vi "Commands.vi"(8 "error in (no error)":errorcluster, 11 "Node Ptr":T1 format="%.0x") -> (0 "error out":errorcluster)   [LabVIEW 2019, in "Diagnostics Addon System Explorer.lvlib"]
uses:
  Diagnostics Addon System Explorer.lvlib
  <vilib>/NI VeriStand/Custom Device API/Custom Device Item Ref.ctl
  Types/FG.Action.ctl
  Addon Shared/SubVIs/Constants.vi
  <vilib>/NI VeriStand/Custom Device API/NI VeriStand - Get Item Property.vi
  <vilib>/NI VeriStand/Custom Device API/Get Item Property (String).vi
  <vilib>/NI VeriStand/Custom Device API/Get Item Property (Variant).vi
  <vilib>/NI VeriStand/Custom Device API/Get Item Property (U32).vi
  <vilib>/NI VeriStand/Custom Device API/Get Item Property (Boolean).vi
  <vilib>/NI/NI VeriStand Advanced SysDef API/SysDef API/SysDef.Property.Set.vi
  <vilib>/NI/NI VeriStand Advanced SysDef API/_SubVIs/SysDef.Property.Set.String.vi
  <vilib>/NI/NI VeriStand Advanced SysDef API/_SubVIs/SysDef.Property.Set.Variant.vi
  <vilib>/NI/NI VeriStand Advanced SysDef API/_SubVIs/SysDef.Property.Set.U32.vi
  <vilib>/NI/NI VeriStand Advanced SysDef API/_SubVIs/SysDef.Property.Set.Boolean.vi
  <vilib>/NI VeriStand/Custom Device API/Custom Device API.lvlib
panel:
  in  "SHDocVw.IWebBrowser":refnum<k7>(container)
  in  "Header":cluster{"Section Name":string}={"Section Name"="Custom Device Item Settings"}
  in  "Description":string
  in  "Name":string
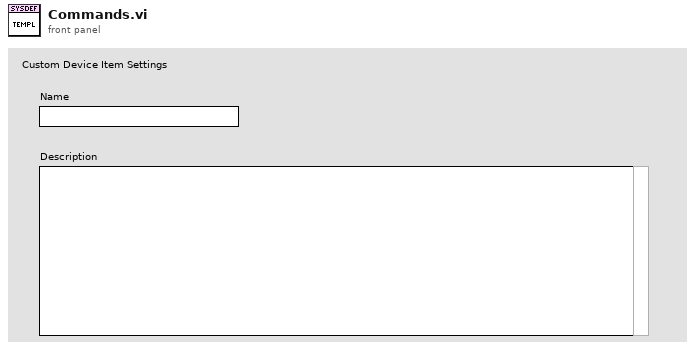
[diagram p1: front panel]
types:
  T1 = typedef "Custom Device API.lvlib/Custom Device Item Ref.ctl" = u64
  T2 = typedef "Diagnostics Addon System Explorer.lvlib/FG.Action.ctl" = enum16{"Get", "Set"}
  T3 = typedef "Diagnostics Addon Shared.lvlib/CAN.ctl" = cluster{"Interface":T4, "Baud Rate":u64, "Diagnostic Protocol":T5, "Transport Protocol":T6, "Transmit ID":u32, "Receive ID":u32, "Transmit Extension":u8, "Receive Extension":u8, "Receive UUDT ID":u32, "Enable Stream":bool, "VW TP Channel ID":u32, "Fill Frame":bool, "Fill Byte":u8, "Termination":bool, "LIN Cluster":refnum<k21>, "NAD":u8, "IO Mode":u32, "Max DLC":u16, "FD Baud Rate":u64, "Timeout":u32}
  T4 = typedef "Diagnostics Addon Shared.lvlib/CAN.Interface.ctl" = string
  T5 = typedef "Diagnostics Addon Shared.lvlib/Protocol.ctl" = enum16{"GMLAN", "KWP-2000", "UDS", "User-Defined"}
  T6 = typedef "Diagnostics Addon Shared.lvlib/Transport.ctl" = enum16{"ISO TP - Normal Mode", "ISO TP - Mixed Mode", "VW TP 2.0", "Diagnostics on IP", "ISO TP LIN"}
  T7 = typedef "Custom Device API.lvlib/Custom Device Item Info.ctl" = cluster{"Name":string, "Is Channel":bool, "GUID":string, "Is Waveform":bool}
  T8 = typedef "Custom Device API.lvlib/Custom Device Commands.ctl" = enum16{"Default", "Item renamed", "Shutdown", "Dynamic button pressed"}
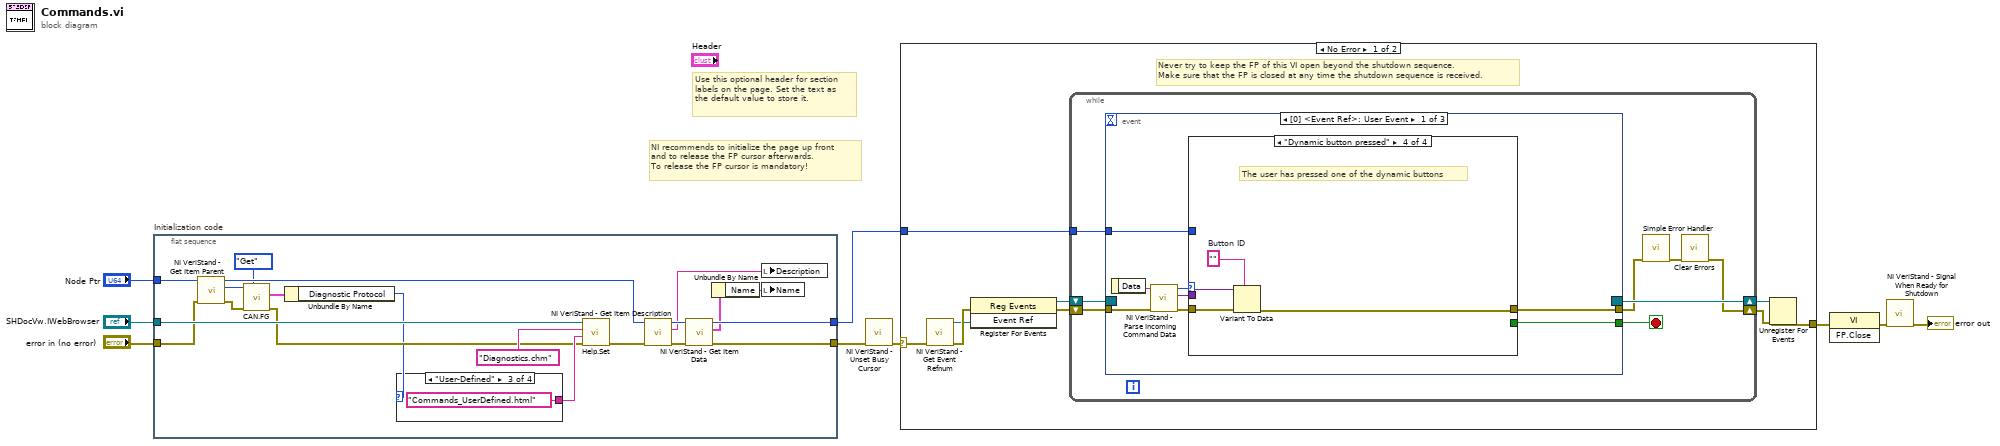
[diagram p0: block diagram]
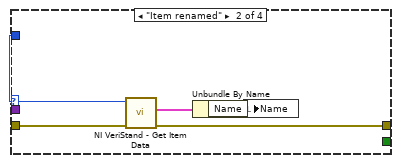
[diagram p3: hidden frame]
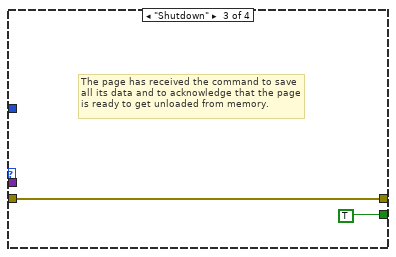
[diagram p4: hidden frame]
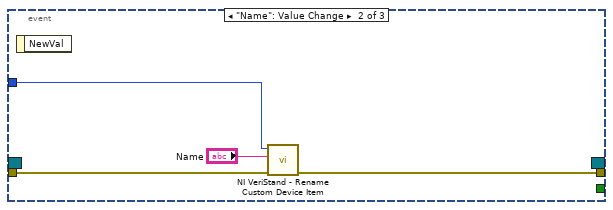
[diagram p5: hidden frame]
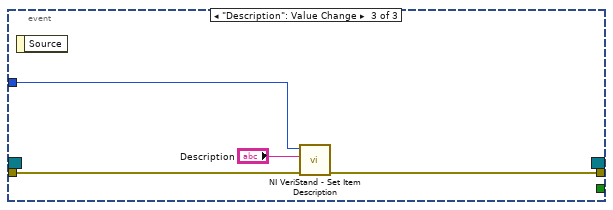
[diagram p6: hidden frame]
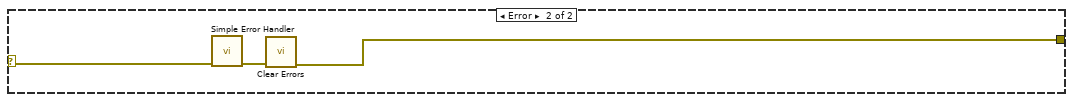
[diagram p7: hidden frame]
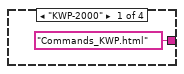
[diagram p8: hidden frame]
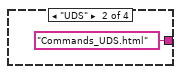
[diagram p9: hidden frame]
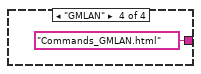
[diagram p10: hidden frame]
diagram:
  # "Use this optional header for section labels on the page. Set the text as the default value to store it."
  # "NI recommends to initialize the page up front\nand to release the FP cursor afterwards.\nTo release the FP cursor is mandatory!"
  n1 = flat-sequence "Initialization code" {
    tunnel: "error in (no error)" -> [w18]
    tunnel: "Node Ptr" -> [w17]
    tunnel: [w23] -> w5
    tunnel: [w29] -> w2
    tunnel: "SHDocVw.IWebBrowser" -> [w19]
    frame #0 {
      n2 = call <vilib>:"NI VeriStand - Get Item Parent.vi"("error in (no error)"=w18, "Item Ref in"=w17) -> ("error out"=w13:errorcluster, "Parent Ref"=w15:T1, "Item Ref out"=w16:T1)  [unwired: 6 in, 1 out]
      n3 = call "CAN.FG.vi"("Action"=FG.Action."Get", "error in (no error)"=w13, "Device Item Ref in"=w15) -> ("error out"=w12:errorcluster, "Diagnostics Basic Configuration"=w11:T3)  [unwired: 6 in, 1 out]
      n4 = Unbundle By Name(w11) -> ("Diagnostic Protocol"=w10:T5)
      n5 = case shown="\"User-Defined\"" w10 {
        tunnel: ["Commands_KWP.html" ("HTML File") "Commands_UDS.html" ("HTML File") "Commands_UserDefined.html" ("HTML File") "Commands_GMLAN.html" ("HTML File")] -> w21
        frame "KWP-2000" {
        }
        frame "UDS" {
        }
        frame "User-Defined" {
        }
        frame "GMLAN" {
        }
      }
      n6 = call "Help.Set.vi"("error in (no error)"=w12, "HTML File"=w21, "Main CHM File"="Diagnostics.chm", "SHDocVw.IWebBrowser2"=w19) -> ("error out"=w20:errorcluster)  [unwired: 7 in]
      n7 = call <vilib>:"NI VeriStand - Get Item Description.vi"("error in (no error)"=w20, "Item Ref in"=w16) -> ("error out"=w26:errorcluster, "Description"=w27:string, "Item Ref out"=w28:T1)  [unwired: 7 out]
      n8 = call <vilib>:"NI VeriStand - Get Item Data.vi"("error in (no error)"=w26, "Item Ref in"=w28) -> ("error out"=w23:errorcluster, "Item Info"=w25:T7, "Item Ref out"=w29:T1)  [unwired: 7 out]
      n9 = Unbundle By Name(w25) -> ("Name"=w24:string)
      n10 = local write "Description"(w27) -> ()
      n11 = local write "Name"(w24) -> ()
    }
  }
  n12 = call <vilib>:"NI VeriStand - Unset Busy Cursor.vi"("error in (no error)"=w5) -> ("error out"=w4:errorcluster)  [unwired: 10 out]
  n13 = case shown="No Error" w4 {
    selector: w4 -> [w34 w81]
    tunnel: [w39 w79] -> w9
    tunnel: w2 -> [w35 _]
    frame No Error {
      # "Never try to keep the FP of this VI open beyond the shutdown sequence.\nMake sure that the FP is closed at any time the shutdown sequence is received."
      n14 = call <vilib>:"NI VeriStand - Get Event Refnum.vi"("error in (no error)"=w34) -> ("error out"=w42:errorcluster, "Event Ref"=w38:refnum<user-event>)  [unwired: 9 out]
      n15 = register-events(error in=w42, w38) -> (reference out=w36:refnum<event-registration>, error out=w37:errorcluster)  [unwired: 1 in]
      n16 = while {
        tunnel: w35 -> [w46]
        shift-right: [w43] -> w40
        shift-left: w37 -> [w49]
        shift-right: [w50] -> w41
        shift-left: w36 -> [w48]
        stop <- w47 stop-if-true
        n17 = event shown="[0] <Event Ref>: User Event" {
          selector: w48 -> [_ _ _]
          dyn-events: [_ _ _] -> w50
          timeout: _ -> [_ _ _]
          tunnel: w49 -> [w58 w74 w77]
          tunnel: [w54 _ _] -> w47
          tunnel: [w53 w73 w76] -> w45
          tunnel: w46 -> [w52 w72 w78]
          event User Event {
            n18 = event-data() -> ("Data"=w57:string)  [unwired: 1 out]
            n19 = call <vilib>:"NI VeriStand - Parse Incoming Command Data.vi"("error in (no error)"=w58, "Incoming data"=w57) -> ("error out"=w56:errorcluster, "Outgoing data"=w51:variant, "Action"=w55:T8)  [unwired: 7 out]
            n20 = case shown="\"Dynamic button pressed\"" w55 {
              tunnel: w56 -> [w59 w64 w65 w70]
              tunnel: [_ _ TRUE _] -> w54
              tunnel: [w59 w61 w65 w67] -> w53
              tunnel: w52 -> [_ w63 _ _]
              tunnel: w51 -> [_ _ _ w69]
              frame "Default", Default {
              }
              frame "Item renamed" {
                n21 = call <vilib>:"NI VeriStand - Get Item Data.vi"("error in (no error)"=w64, "Item Ref in"=w63) -> ("error out"=w61:errorcluster, "Item Info"=w62:T7)  [unwired: 8 out]
                n22 = Unbundle By Name(w62) -> ("Name"=w60:string)
                n23 = local write "Name"(w60) -> ()
              }
              frame "Shutdown" {
                # "The page has received the command to save all its data and to acknowledge that the page is ready to get unloaded from memory."
              }
              frame "Dynamic button pressed" {
                w68 = ""  # Button ID
                # "The user has pressed one of the dynamic buttons"
                n24 = Variant To Data(error in=w70, type=w68, Variant=w69) -> (error out=w67:errorcluster)  [unwired: 1 out]
              }
            }
          }
          event "Name": Value Change {
            n25 = event-data() -> ()  [unwired: 2 out]
            n26 = call <vilib>:"NI VeriStand - Rename Custom Device Item.vi"("error in (no error)"=w74, "New Name"="Name", "Item Ref in"=w72) -> ("error out"=w73:errorcluster)  [unwired: 1 in, 7 out]
          }
          event "Description": Value Change {
            n27 = event-data() -> ()  [unwired: 2 out]
            n28 = call <vilib>:"NI VeriStand - Set Item Description.vi"("error in (no error)"=w77, "Description"="Description", "Item Ref in"=w78) -> ("error out"=w76:errorcluster)  [unwired: 8 out]
          }
        }
        n29 = call <vilib>:"Simple Error Handler.vi"("error in (no error)"=w45) -> ("error out"=w44:errorcluster)  [unwired: 1 in, 7 out]
        n30 = call <vilib>:"Clear Errors.vi"("error in (no error)"=w44) -> ("error out"=w43:errorcluster)  [unwired: 1 in, 5 out]
      }
      n31 = Unregister For Events(event registration refnum=w41, error in=w40) -> (error out=w39:errorcluster)
    }
    frame Error {
      n32 = call <vilib>:"Simple Error Handler.vi"("error in (no error)"=w81) -> ("error out"=w80:errorcluster)  [unwired: 1 in, 7 out]
      n33 = call <vilib>:"Clear Errors.vi"("error in (no error)"=w80) -> ("error out"=w79:errorcluster)  [unwired: 1 in, 5 out]
    }
  }
  n34 = invoke class="VI" method="FP.Close"(error in=w9) -> (error out=w8:errorcluster)  [unwired: 2 in, 2 out]
  n35 = call <vilib>:"NI VeriStand - Signal When Ready for Shutdown.vi"("error in (no error)"=w8) -> ("error out"=→"error out":errorcluster)  [unwired: 10 out]
